vi "Teleop.vi"(10 "Match Info":T1={"Autonomous Elapsed Seconds"=0.0, "TeleOp Elapsed Seconds"=0.0, "Disabled Elapsed Seconds"=0.0, "Visited Autonomous"=FALSE, "Visited TeleOp"=FALSE, "Visited Disabled"=FALSE, "Autonomous Settings"={"Autonomous Style"=enum."Independent", "VI Refnum"=refnum}}, 11 "Call Context":T2) -> ()   [LabVIEW 2023]
doc: "This VI is called for each enabled TeleOp packet received from the DS. It is typically used to read from joysticks and other inputs and update I/O or setpoints for timed control loops. It should complete and return within 20 milliseconds or risk missing DS packets."
uses:
  <vilib>/Rock Robotics/WPI/DriverStation/WPI_DriverStationDerivedRobotMode.ctl
  <vilib>/Rock Robotics/WPI/DriverStation/WPI_DriverStationMatch Info.ctl
  <vilib>/Rock Robotics/WPI/Joystick/XBox Buttons Indexer.ctl
  <vilib>/Rock Robotics/WPI/Joystick/XBox Axes Indexer.ctl
  Climber/Implementation/Climber Operations.ctl
  AimTIFKATS/Implementation/AimTIFKATS Operations.ctl
  Swerve/Implementation/Swerve Setpoints2.ctl
  Swerve/Implementation/Swerve Operations.ctl
  Undertake/Implementation/Undertake Operations.ctl
  TIFKATS/Implementation/TIFKATS Operations.ctl
  <vilib>/Rock Robotics/WPI/Utilities/WPI_GetSetVariantRefNum.vi
  <vilib>/Rock Robotics/Network Tables/NT Write Boolean Array.vi
  <vilib>/Rock Robotics/Network Tables/NT Write Numeric Array.vi
  <vilib>/Rock Robotics/Network Tables/NT Read Boolean.vi
  <vilib>/Rock Robotics/Network Tables/NT Write Number.vi
  Framework/Robot Global Data.vi
  <vilib>/Rock Robotics/Network Tables/NT Read Float.vi
panel:
  out "TIFKATS Angle":dbl
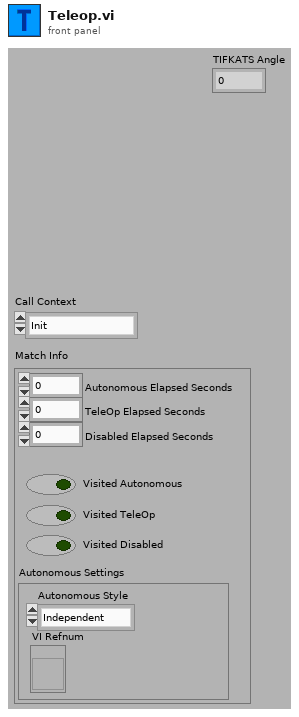
[diagram p1: front panel]
types:
  T1 = typedef "WPI_DriverStationMatch Info.ctl" = cluster{"Autonomous Elapsed Seconds":dbl, "TeleOp Elapsed Seconds":dbl, "Disabled Elapsed Seconds":dbl, "Visited Autonomous":bool, "Visited TeleOp":bool, "Visited Disabled":bool, "Autonomous Settings":cluster{"Autonomous Style":enum16{"Iterative", "Independent"}, "VI Refnum":refnum<vi>}}
  T2 = typedef "WPI_DriverStationDerivedRobotMode.ctl" = enum16{"Init", "Execute", "Stop"}
  T3 = typedef "XBox Buttons Indexer.ctl" = enum16{"A", "B", "X", "Y", "Left Bumper", "Right Bumper", "Back", "Start", "Left Joystick", "Right Joystick"}
  T4 = typedef "XBox Axes Indexer.ctl" = enum16{"Left X", "Left Y", "Left Trigger", "Right Trigger", "Right X", "Right Y"}
  T5 = typedef "WPI_JoystickDevRef.ctl" = cluster{"Device":T6}
  T6 = typedef "WPI_JoystickDeviceEnum.ctl" = enum16{"USB 0", "USB 1", "USB 2", "USB 3", "USB 4", "USB 5"}
  T7 = typedef "Climber Operations.ctl" = enum16{"Reserve", "Read Current", "Immediate", "Move up", "Move down", "Stop"}
  T8 = typedef "AimTIFKATS Operations.ctl" = enum16{"Reserve", "Read Current", "Immediate", "Angle up", "Angle down", "Angle to angle", "Stop rotate"}
  T9 = typedef "TIFKATS Operations.ctl" = enum16{"Reserve", "Read Current", "Immediate", "Load", "Shoot", "Intake", "Spit", "Stop All"}
  T10 = typedef "WPI_MotorControlDeviceRef.ctl" = cluster{"DeviceStatus":errorcluster, "Type":T11, "PWM":cluster{"PWM Channel":T12, "DeadBand":T13}, "CAN":cluster{"Device Number":u8, "SetOutput VI Ref":variant, "GetOutput VI Ref":variant, "Enable VI Ref":variant, "Disable VI Ref":variant, "Data":variant}, "Invert":bool, "DIO PWM":cluster{"PWM \"Enable\" Channel":T12, "DIOChannel":T14, "PWM Rate":dbl}}
  T11 = typedef "WPI_MotorControlType.ctl" = enum16{"PWM", "CAN", "DIO PWM"}
  T12 = typedef "FPGA_DIOPWMChannel.ctl" = enum8{"PWM 0", "PWM 1", "PWM 2", "PWM 3", "PWM 4", "PWM 5", "PWM 6", "PWM 7", "PWM 8", "PWM 9", "PWM MXP 0", "PWM MXP 1", "PWM MXP 2", "PWM MXP 3", "PWM MXP 4", "PWM MXP 5", "PWM MXP 6", "PWM MXP 7", "PWM MXP 8", "PWM MXP 9", "Invalid"}
  T13 = typedef "WPI_PWMDeadband.ctl" = cluster{"Name":string, "maxPositivePwm":i32, "minPositivePwm":i32, "centerPwm":i32, "maxNegativePwm":i32, "minNegativePwm":i32, "angularRange":u16}
  T14 = typedef "FPGA_DIOChannel.ctl" = enum8{"DIO 0", "DIO 1", "DIO 2", "DIO 3", "DIO 4", "DIO 5", "DIO 6", "DIO 7", "DIO 8", "DIO 9", "DIO MXP 0", "DIO MXP 1", "DIO MXP 2", "DIO MXP 3", "DIO MXP 4", "DIO MXP 5", "DIO MXP 6", "DIO MXP 7", "DIO MXP 8", "DIO MXP 9", "DIO MXP 10", "DIO MXP 11", "DIO MXP 12", "DIO MXP 13", "DIO MXP 14", "DIO MXP 15", "SPI Port CS1", "SPI Port CS2", "SPI Port CS3", "SPI Port MISO", "SPI Port MOSI", "Invalid"}
  T15 = typedef "Undertake Operations.ctl" = enum16{"Reserve", "Read Current", "Immediate", "Onn", "Offf", "Reject"}
  T16 = typedef "ADIS16470 Device Reference.ctl" = cluster{"DevStatus":errorcluster, "Hardware Config":T17, "Calibration Complete":refnum<notifier>, "Status Reference":refnum<data-value>, "Data Reference":refnum<data-value>, "Sychronous Process VI":T20, "Cmd FIFO":refnum<k33>, "Source":T21, "Data FIFO":refnum<k33>, "Calibration Time (ms)":u32, "Data Reference":refnum<data-value>}
  T17 = typedef "ADIS16470 Hardware Configuration.ctl" = cluster{"SPI Clock Rate (Hz)":dbl, "IMU SPI Mode (3)":T18, "IMU Reset Pin":T14, "IMU SPI Bus":T19, "IMU Data Ready Pin":T14, "Stall Config":cluster{"Pow2BytesPerRead":u8, "StallTicks":u16, "CsToSclkTicks":u8}}
  T18 = typedef "WPI_SPIMode.ctl" = enum16{"Mode 0 (Clk Idle Low,Sample on Leading)", "Mode 1 (Clk Idle Low,Sample on Trailing)", "Mode 2 (Clk Idle High,Sample on Leading)", "Mode 3 (Clk Idle High,Sample on Trailing)"}
  T19 = typedef "spi_bus.ctl" = enum16{"SPI On-Board, CS0", "SPI On-Board, CS1", "SPI On-Board, CS2", "SPI On-Board, CS3", "SPI MXP", "Invalid"}
  T20 = typedef "ADIS16470 Process.ctl" = refnum<vi>
  T21 = typedef "FPGA_CounterEncoderSourceConvertionLVSourceType.ctl" = cluster{"DevStatus":errorcluster, "AnalogTriggerMode?":bool, "DigitalMode":cluster{"DIO Channel":T22}, "AnalogTriggerMode":cluster{"AnalogTriggerIndex":T23, "OutputType":T24}}
  T22 = typedef "FPGA_DIODigitalSourceChannel.ctl" = enum8{"DIO 0", "DIO 1", "DIO 2", "DIO 3", "DIO 4", "DIO 5", "DIO 6", "DIO 7", "DIO 8", "DIO 9", "DIO MXP 0", "DIO MXP 1", "DIO MXP 2", "DIO MXP 3", "DIO MXP 4", "DIO MXP 5", "DIO MXP 6", "DIO MXP 7", "DIO MXP 8", "DIO MXP 9", "DIO MXP 10", "DIO MXP 11", "DIO MXP 12", "DIO MXP 13", "DIO MXP 14", "DIO MXP 15", "SPI Port CS1", "SPI Port CS2", "SPI Port CS3", "SPI Port MISO", "SPI Port MOSI", "Disabled"}
  T23 = typedef "FPGA_AnalogTriggerIndex.ctl" = enum8{"Trig 0", "Trig 1", "Trig 2", "Trig 3", "Trig 4", "Trig 5", "Trig 6", "Trig 7", "Invalid"}
  T24 = typedef "FPGA_AnalogTriggerOutType.ctl" = enum16{"InWindow", "TriggerState", "Rising", "Falling"}
  T25 = typedef "ADIS16470 Data.ctl" = cluster{"XAngle":dbl, "YAngle":dbl, "ZAngle":dbl}
  T26 = cluster{"proportional gain (Kp)":dbl, "integral time (Ki)":dbl, "derivative time (Kd)":dbl}
  T27 = typedef "Swerve Setpoints2.ctl" = cluster{"Operation":T28, "Gyro":dbl, "FWD":dbl, "STR":dbl, "X rotate":dbl, "Y rotate":dbl, "Time":dbl, "Distance":dbl, "Right Trigger":dbl, "Angle":dbl, "Start Angle":dbl, "Tag ID":dbl, "Start Positions":dbl[]}
  T28 = typedef "Swerve Operations.ctl" = enum16{"Reserve", "Read Current", "Immediate", "Stop", "Balance", "Direct  Joystick Drive", "Joystick Drive", "Drive for Distance", "Drive for Time", "Turn to Angle", "Drive to Angle(Time)", "Drive to Angle(Distance)", "Look At Cone", "Look At Cube", "Move To Tape", "Move To Tag"}
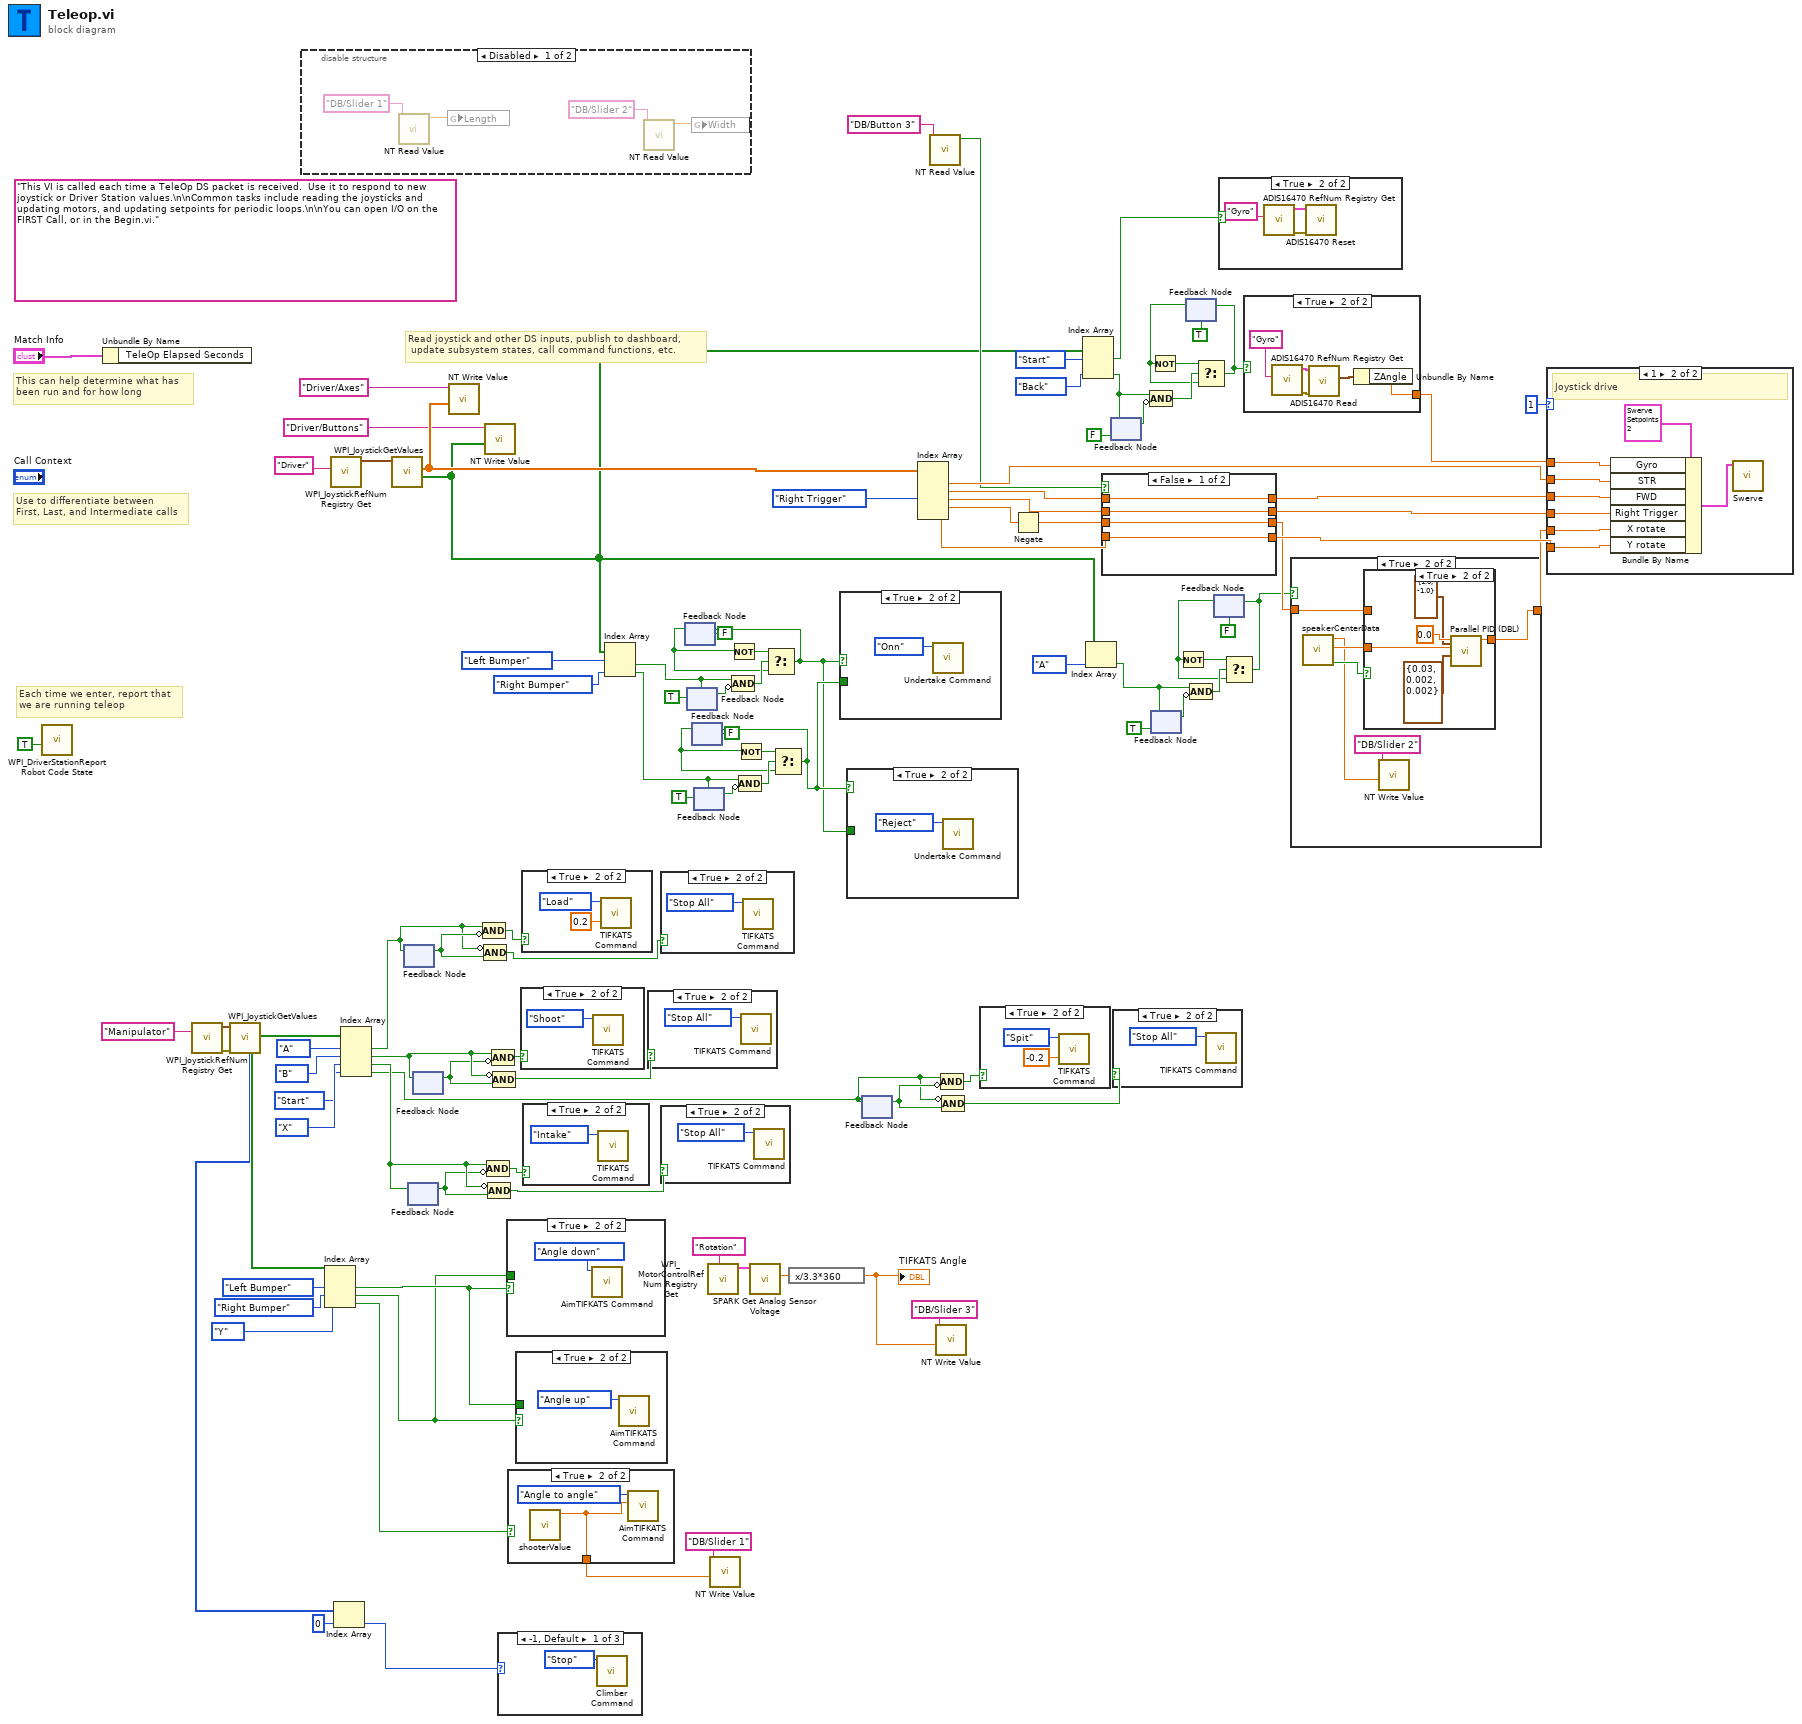
[diagram p0: block diagram]
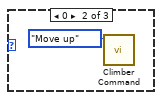
[diagram p2: hidden frame]
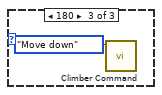
[diagram p3: hidden frame]
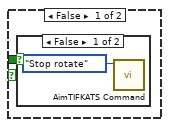
[diagram p4: hidden frame]
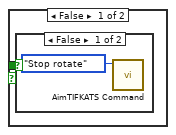
[diagram p6: hidden frame]
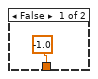
[diagram p8: hidden frame]
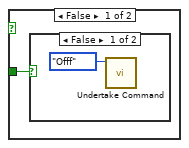
[diagram p17: hidden frame]
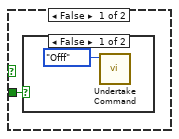
[diagram p19: hidden frame]
diagram:
  (unwired) "This VI is called each time a TeleOp DS packet is received.  Use it to respond to new joystick or Driver Station values.\n\nCommon tasks include reading the joysticks and updating motors, and updating setpoints for periodic loops.\n\nYou can open I/O on the FIRST Call, or in the Begin.vi."
  # "Read joystick and other DS inputs, publish to dashboard,\n update subsystem states, call command functions, etc."
  # "Each time we enter, report that\nwe are running teleop"
  # "Use to differentiate between\nFirst, Last, and Intermediate calls"
  # "This can help determine what has\nbeen run and for how long"
  n1 = call <vilib>:"WPI_DriverStationReport Robot Code State.vi"("TeleOp"=TRUE ("Autonomous")) -> ()  [unwired: 10 in, 1 out]
  n2 = Unbundle By Name("Match Info") -> ()  [unwired: 1 out]
  n3 = call <vilib>:"WPI_JoystickRefNum Registry Get.vi"("refnum name"="Manipulator") -> ("error out"=w69:errorcluster, "JoystickDevRef"=w70:T5)  [unwired: 1 in, 8 out]
  n4 = call <vilib>:"WPI_JoystickGetValues.vi"("error in (no error)"=w69, "JoystickDevRef"=w70) -> ("Buttons"=w4:bool[], "POVs"=w3:i16[])  [unwired: 5 in, 3 out]
  n5 = disable-structure shown="Disabled" {
    frame Disabled {
      n6 = call-poly <vilib>:"NT Read Value.vi"("name"="DB/Slider 1") -> ("value"=w105:dbl)  [unwired: 8 in, 2 out]
      n7 = global write "Robot Global Data.vi" "Length"(w105) -> ()
      n8 = call-poly <vilib>:"NT Read Value.vi"("name"="DB/Slider 2") -> ("value"=w103:dbl)  [unwired: 8 in, 2 out]
      n9 = global write "Robot Global Data.vi" "Width"(w103) -> ()
    }
    frame Enabled {
    }
  }
  n10 = Index Array(array=w4, index #1=XBox_Buttons_Indexer."Left Bumper" ("XBox Buttons"), index #2=XBox_Buttons_Indexer."Right Bumper" ("XBox Buttons"), index #3=XBox_Buttons_Indexer."Y" ("XBox Buttons")) -> (element #1=w28:bool, element #2=w27:bool, element #3=w61:bool)
  n11 = call <vilib>:"WPI_JoystickRefNum Registry Get.vi"("refnum name"="Driver") -> ("JoystickDevRef"=w99:T5)  [unwired: 1 in, 9 out]
  n12 = Index Array(array=w3, index=0) -> (element=w1:i16)
  n13 = Index Array(array=w4, index #1=XBox_Buttons_Indexer."A" ("XBox Buttons"), index #2=XBox_Buttons_Indexer."B" ("XBox Buttons"), index #3=XBox_Buttons_Indexer."X" ("XBox Buttons"), index #4=XBox_Buttons_Indexer."Start" ("XBox Buttons")) -> (element #1=w9:bool, element #2=w65:bool, element #3=w48:bool, element #4=w13:bool)
  n14 = call <vilib>:"WPI_JoystickGetValues.vi"("JoystickDevRef"=w99) -> ("Buttons"=w47:bool[], "Axes"=w98:dbl[])  [unwired: 6 in, 3 out]
  n15 = feedback #1() -> (w10:bool)  [unwired: 1 in]
  n16 = feedback-in #1(w9) -> ()
  n17 = feedback #2() -> (w20:bool)  [unwired: 1 in]
  n18 = feedback-in #2(w48) -> ()
  n19 = feedback #3() -> (w22:bool)  [unwired: 1 in]
  n20 = feedback-in #3(w65) -> ()
  n21 = call-poly <vilib>:"NT Write Value.vi"("value"=w98, "name"="Driver/Axes" ("Name")) -> ()  [unwired: 9 in, 1 out]
  n22 = Compound Arithmetic op=AND(w9, invert w10) -> (w8:bool)
  n23 = Compound Arithmetic op=AND(invert w9, w10) -> (w7:bool)
  n24 = call-poly <vilib>:"NT Write Value.vi"("value"=w47, "name"="Driver/Buttons" ("Name")) -> ()  [unwired: 9 in, 1 out]
  n25 = Compound Arithmetic op=AND(w48, invert w20) -> (w19:bool)
  n26 = Compound Arithmetic op=AND(invert w48, w20) -> (w18:bool)
  n27 = Compound Arithmetic op=AND(w65, invert w22) -> (w23:bool)
  n28 = Compound Arithmetic op=AND(invert w65, w22) -> (w21:bool)
  n29 = case shown="-1, Default" w1 {
    frame -1, Default {
      n30 = call "Climber Command.vi"("Operation"=Climber_Operations."Stop") -> ()  [unwired: 9 in, 1 out]
    }
    frame 0 {
      n31 = call "Climber Command.vi"("Operation"=Climber_Operations."Move up") -> ()  [unwired: 9 in, 1 out]
    }
    frame 180 {
      n32 = call "Climber Command.vi"("Operation"=Climber_Operations."Move down") -> ()  [unwired: 9 in, 1 out]
    }
  }
  n33 = case shown="True" w28 {
    tunnel: w27 -> [w110 _]
    frame False {
      n34 = case shown="False" w110 {
        frame False {
          n35 = call "AimTIFKATS Command.vi"("Operation"=AimTIFKATS_Operations."Stop rotate") -> ()  [unwired: 9 in, 1 out]
        }
        frame True {
        }
      }
    }
    frame True {
      n36 = call "AimTIFKATS Command.vi"("Operation"=AimTIFKATS_Operations."Angle down") -> ()  [unwired: 9 in, 1 out]
    }
  }
  n37 = case shown="True" w61 {
    tunnel: [-1.0 ("Interpolated value") w114] -> w5
    frame False {
    }
    frame True {
      n38 = call "shooterValue.vi"() -> ("Interpolated value"=w114:dbl)  [unwired: 11 in]
      n39 = call "AimTIFKATS Command.vi"("Operation"=AimTIFKATS_Operations."Angle to angle", "Setpoint"=w114) -> ()  [unwired: 8 in, 1 out]
    }
  }
  n40 = case shown="True" w27 {
    tunnel: w28 -> [w116 _]
    frame False {
      n41 = case shown="False" w116 {
        frame False {
          n42 = call "AimTIFKATS Command.vi"("Operation"=AimTIFKATS_Operations."Stop rotate") -> ()  [unwired: 9 in, 1 out]
        }
        frame True {
        }
      }
    }
    frame True {
      n43 = call "AimTIFKATS Command.vi"("Operation"=AimTIFKATS_Operations."Angle up") -> ()  [unwired: 9 in, 1 out]
    }
  }
  n44 = case shown="True" w23 {
    frame False {
    }
    frame True {
      n45 = call "TIFKATS Command.vi"("Operation"=TIFKATS_Operations."Shoot") -> ()  [unwired: 10 in, 1 out]
    }
  }
  n46 = case shown="True" w8 {
    frame False {
    }
    frame True {
      n47 = call "TIFKATS Command.vi"("Setpoint"=0.2, "Operation"=TIFKATS_Operations."Load") -> ()  [unwired: 9 in, 1 out]
    }
  }
  n48 = case shown="True" w19 {
    frame False {
    }
    frame True {
      n49 = call "TIFKATS Command.vi"("Operation"=TIFKATS_Operations."Intake") -> ()  [unwired: 10 in, 1 out]
    }
  }
  n50 = Index Array(array=w47, index #1=XBox_Buttons_Indexer."Left Bumper" ("XBox Buttons"), index #2=XBox_Buttons_Indexer."Right Bumper" ("XBox Buttons")) -> (element #1=w38:bool, element #2=w31:bool)
  n51 = case shown="True" w21 {
    frame False {
    }
    frame True {
      n52 = call "TIFKATS Command.vi"("Operation"=TIFKATS_Operations."Stop All") -> ()  [unwired: 10 in, 1 out]
    }
  }
  n53 = case shown="True" w7 {
    frame False {
    }
    frame True {
      n54 = call "TIFKATS Command.vi"("Operation"=TIFKATS_Operations."Stop All") -> ()  [unwired: 10 in, 1 out]
    }
  }
  n55 = case shown="True" w18 {
    frame False {
    }
    frame True {
      n56 = call "TIFKATS Command.vi"("Operation"=TIFKATS_Operations."Stop All") -> ()  [unwired: 10 in, 1 out]
    }
  }
  n57 = feedback #4(FALSE) -> (w39:bool)
  n58 = feedback #5(TRUE) -> (w44:bool)
  n59 = feedback-in #5(w38) -> ()
  n60 = feedback #6(FALSE) -> (w32:bool)
  n61 = feedback #7(TRUE) -> (w37:bool)
  n62 = feedback-in #7(w31) -> ()
  n63 = call <vilib>:"WPI_MotorControlRefNum Registry Get.vi"("refnum name"="Rotation") -> ("MotorControlDevRef"=w25:T10)  [unwired: 9 in, 1 out]
  n64 = call-poly <vilib>:"NT Write Value.vi"("value"=w5, "name"="DB/Slider 1") -> ()  [unwired: 9 in, 1 out]
  n65 = Not(x=w39) -> (.not. x?=w42:bool)
  n66 = Compound Arithmetic op=AND(w38, invert w44) -> (w40:bool)
  n67 = Not(x=w32) -> (.not. x?=w35:bool)
  n68 = Compound Arithmetic op=AND(w31, invert w37) -> (w33:bool)
  n69 = call <vilib>:"SPARK Get Analog Sensor Voltage.vi"("MotorControlDevRef in"=w25) -> ("Analog Sensor Voltage"=w24:dbl)  [unwired: 7 in, 3 out]
  n70 = Select(t=w42, s=w40, f=w39) -> (s? t:f=w29:bool)
  n71 = feedback-in #4(w29) -> ()
  n72 = Select(t=w35, s=w33, f=w32) -> (s? t:f=w30:bool)
  n73 = feedback-in #6(w30) -> ()
  n74 = expression code="x/3.3*360"(w24) -> (w11:dbl)
  "TIFKATS Angle" <- w11
  n75 = case shown="True" w29 {
    tunnel: w30 -> [w126 _]
    frame False {
      n76 = case shown="False" w126 {
        frame False {
          n77 = call "Undertake Command.vi"("Operation"=Undertake_Operations."Offf") -> ()  [unwired: 9 in, 1 out]
        }
        frame True {
        }
      }
    }
    frame True {
      n78 = call "Undertake Command.vi"("Operation"=Undertake_Operations."Onn") -> ()  [unwired: 9 in, 1 out]
    }
  }
  n79 = case shown="True" w30 {
    tunnel: w29 -> [w129 _]
    frame False {
      n80 = case shown="False" w129 {
        frame False {
          n81 = call "Undertake Command.vi"("Operation"=Undertake_Operations."Offf") -> ()  [unwired: 9 in, 1 out]
        }
        frame True {
        }
      }
    }
    frame True {
      n82 = call "Undertake Command.vi"("Operation"=Undertake_Operations."Reject") -> ()  [unwired: 9 in, 1 out]
    }
  }
  n83 = feedback #8() -> (w15:bool)  [unwired: 1 in]
  n84 = feedback-in #8(w13) -> ()
  n85 = Index Array(array=w98, index #3=XBox_Axes_Indexer."Right Trigger" ("XBox Axes")) -> (element #1=w95:dbl, element #2=w92:dbl, element #3=w90:dbl, element #4=w75:dbl, element #5=w87:dbl)  [unwired: 4 in]
  n86 = call-poly <vilib>:"NT Read Value.vi"("name"="DB/Button 3") -> ("value"=w93:bool)  [unwired: 8 in, 2 out]
  n87 = call-poly <vilib>:"NT Write Value.vi"("value"=w11, "name"="DB/Slider 3") -> ()  [unwired: 9 in, 1 out]
  n88 = Compound Arithmetic op=AND(w13, invert w15) -> (w17:bool)
  n89 = Compound Arithmetic op=AND(invert w13, w15) -> (w16:bool)
  n90 = case shown="True" w17 {
    frame False {
    }
    frame True {
      n91 = call "TIFKATS Command.vi"("Setpoint"=-0.2, "Operation"=TIFKATS_Operations."Spit") -> ()  [unwired: 9 in, 1 out]
    }
  }
  n92 = Negate(x=w75) -> (-x=w88:dbl)
  n93 = Index Array(array=w47, index #1=XBox_Buttons_Indexer."Start" ("XBox Buttons"), index #3=XBox_Buttons_Indexer."Back" ("XBox Buttons")) -> (element #1=w72:bool, element #3=w84:bool)  [unwired: 1 in, 1 out]
  n94 = Index Array(array=w47, index=XBox_Buttons_Indexer."A" ("XBox Buttons")) -> (element=w53:bool)
  n95 = case shown="False" w93 {
    tunnel: w92 -> [w137 w146]
    tunnel: [w137 w142] -> w91
    tunnel: w90 -> [w136 w145]
    tunnel: [w136 w141] -> w89
    tunnel: w88 -> [w135 w144]
    tunnel: [w135 w140] -> w52
    tunnel: w87 -> [w134 w143]
    tunnel: [w134 w139] -> w86
    frame False {
    }
    frame True {
      w138 = 0.7 ("x")
      n96 = Multiply(x=w138, y=w145) -> (x*y=w141:dbl)
      n97 = Multiply(x=w138, y=w144) -> (x*y=w140:dbl)
      n98 = Multiply(x=w138, y=w146) -> (x*y=w142:dbl)
      n99 = Multiply(x=w138, y=w143) -> (x*y=w139:dbl)
    }
  }
  n100 = feedback-in #9(w84) -> ()
  n101 = feedback #9(FALSE) -> (w83:bool)
  n102 = case shown="True" w16 {
    frame False {
    }
    frame True {
      n103 = call "TIFKATS Command.vi"("Operation"=TIFKATS_Operations."Stop All") -> ()  [unwired: 10 in, 1 out]
    }
  }
  n104 = Compound Arithmetic op=AND(w84, invert w83) -> (w82:bool)
  n105 = feedback #10(TRUE) -> (w59:bool)
  n106 = feedback-in #10(w53) -> ()
  n107 = feedback #11(TRUE) -> (w80:bool)
  n108 = Not(x=w80) -> (.not. x?=w81:bool)
  n109 = Compound Arithmetic op=AND(w53, invert w59) -> (w55:bool)
  n110 = Select(t=w81, s=w82, f=w80) -> (s? t:f=w79:bool)
  n111 = feedback-in #11(w79) -> ()
  n112 = feedback #12(FALSE) -> (w54:bool)
  n113 = Not(x=w54) -> (.not. x?=w57:bool)
  n114 = case shown="True" w72 {
    frame False {
    }
    frame True {
      n115 = call <vilib>:"ADIS16470 RefNum Registry Get.vi"("refnum name"="Gyro") -> ("error out"=w150:errorcluster, "ADIS16470DevRef out"=w149:T16)  [unwired: 9 in]
      n116 = call <vilib>:"ADIS16470 Reset.vi"("error in (no error)"=w150, "ADIS16470DevRef"=w149) -> ()  [unwired: 8 in, 2 out]
    }
  }
  n117 = Select(t=w57, s=w55, f=w54) -> (s? t:f=w51:bool)
  n118 = feedback-in #12(w51) -> ()
  n119 = case shown="True" w79 {
    tunnel: [0.0 ("ZAngle") w156] -> w49
    frame False {
    }
    frame True {
      n120 = call <vilib>:"ADIS16470 RefNum Registry Get.vi"("refnum name"="Gyro") -> ("error out"=w153:errorcluster, "ADIS16470DevRef out"=w154:T16)  [unwired: 9 in]
      n121 = call <vilib>:"ADIS16470 Read.vi"("error in (no error)"=w153, "ADIS16470DevRef"=w154) -> ("ADIS16470 Value"=w155:T25)  [unwired: 6 in, 3 out]
      n122 = Unbundle By Name(w155) -> ("ZAngle"=w156:dbl)
    }
  }
  n123 = case shown="True" w51 {
    tunnel: w52 -> [w157 w160]
    tunnel: [w157 w162] -> w50
    frame False {
    }
    frame True {
      n124 = call "speakerCenterData.vi"() -> ("DistanceToTarget (Inch)"=w158:dbl, "Target Yaw"=w163:dbl, "Target?"=w161:bool)  [unwired: 7 in, 1 out]
      n125 = case shown="True" w161 {
        tunnel: w163 -> [_ w168]
        tunnel: [w164 w165] -> w162
        tunnel: w160 -> [w164 _]
        frame False {
        }
        frame True {
          n126 = call <vilib>:"Parallel PID (DBL).vi"("output range"=cluster{"high":dbl, "low":dbl} {"high"=1.0, "low"=-1.0}, "PID gains"=T26 {"proportional gain (Kp)"=0.03, "integral time (Ki)"=0.002, "derivative time (Kd)"=0.002}, "process variable"=w168, "setpoint"=0.0) -> ("output"=w165:dbl)  [unwired: 4 in, 3 out]
        }
      }
      n127 = call-poly <vilib>:"NT Write Value.vi"("value"=w158, "name"="DB/Slider 2") -> ()  [unwired: 9 in, 1 out]
    }
  }
  n128 = case shown="1" 1 {
    tunnel: w49 -> [_ w175]
    tunnel: w89 -> [_ w174]
    tunnel: w50 -> [_ w173]
    tunnel: w91 -> [_ w172]
    tunnel: w95 -> [_ w171]
    tunnel: w86 -> [_ w170]
    frame 0, Default {
    }
    frame 1 {
      # "Joystick drive"
      n129 = Bundle By Name(cluster=T27 {"Operation"=enum."Joystick Drive", "Gyro"=0.0, "FWD"=0.0, "STR"=0.0, "X rotate"=0.0, "Y rotate"=0.0, "Time"=0.0, "Distance"=0.0, "Right Trigger"=0.0, "Angle"=0.0, "Start Angle"=0.0, "Tag ID"=0.0, "Start Positions"=[]} ("SubSystem Data"), "Gyro"=w175, "STR"=w171, "FWD"=w172, "Right Trigger"=w174, "X rotate"=w173, "Y rotate"=w170) -> (w176:T27)
      n130 = call "Swerve.vi"("SubSystem Data"=w176) -> ()  [unwired: 10 in, 1 out]
    }
  }
